vi "01TRM800.vi"() -> ()   [LabVIEW 2020]
uses:
  <vilib>/Instr/_visa.llb/VISA Configure Serial Port (Instr).vi
panel:
  out "error out":errorcluster
  out "String":string
  in  "stop":bool
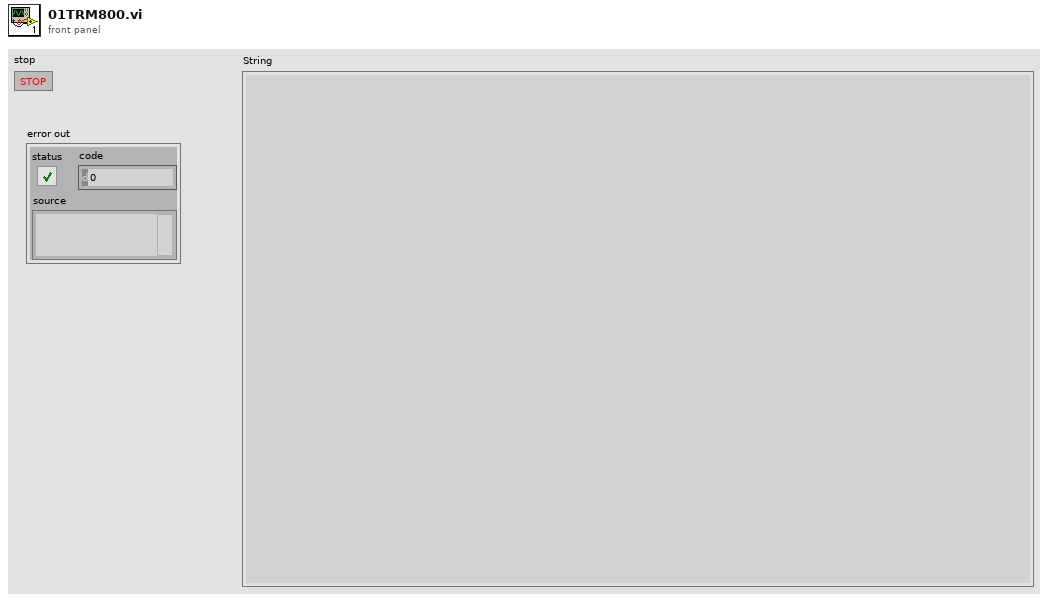
[diagram p1: front panel]
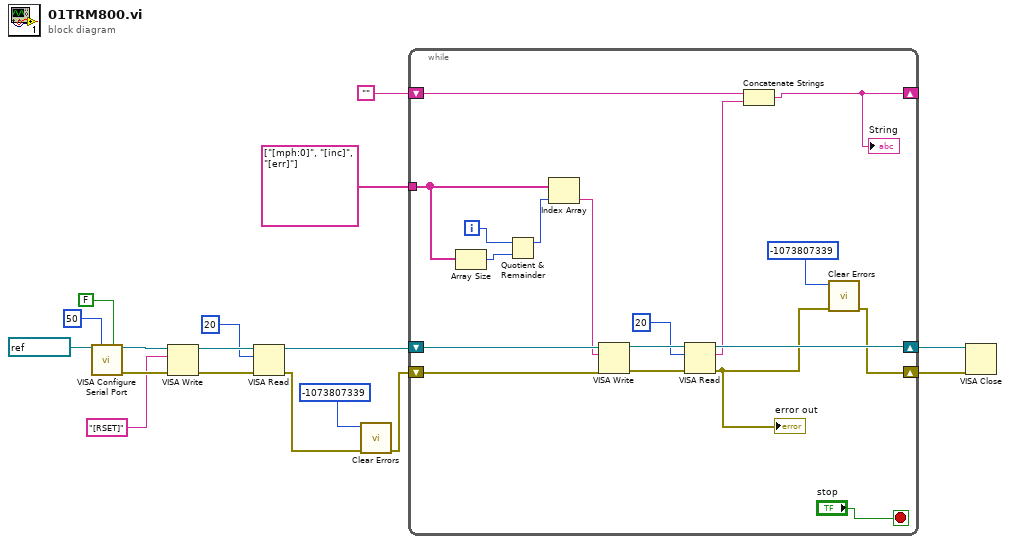
[diagram p0: block diagram]
diagram:
  n1 = call-poly "VISA Configure Serial Port"("VISA resource name"=refnum<visa-resource-name> "COM7", "timeout (10sec)"=u32 50, "Enable Termination\nChar (T)"=FALSE ("Enable Termination\nChar (T)")) -> ("VISA resource name out"=w7:refnum<visa-resource-name>, "error out"=w6:errorcluster)  [unwired: 11 in]
  n2 = VISA Write(VISA resource name=w7, write buffer="[RSET]", error in (no error)=w6) -> (VISA resource name out=w9:refnum<visa-resource-name>, error out=w10:errorcluster)  [unwired: 1 out]
  n3 = VISA Read(VISA resource name=w9, byte count=u32 20, error in (no error)=w10) -> (VISA resource name out=w5:refnum<visa-resource-name>, error out=w3:errorcluster)  [unwired: 2 out]
  n4 = call <vilib>:"Clear Errors.vi"("error in (no error)"=w3, "specific error code to clear (0: all)"=-1073807339) -> ("error out"=w2:errorcluster)  [unwired: 4 in, 1 out]
  n5 = while {
    shift-right: [w24] -> w13
    shift-left: w5 -> [w35]
    shift-right: [w22] -> w12
    shift-left: w2 -> [w30]
    tunnel: string[] ["[mph:0]", "[inc]", "[err]"] -> [w34]
    shift-right: [w18] -> _
    shift-left: "" -> [w20]
    i -> [w32]
    stop <- "stop" stop-if-true
    n6 = Array Size(array=w34) -> (size(s)=w33:i32)
    n7 = Quotient & Remainder(x=w32, y=w33) -> (x-y*floor(x/y)=w31:i32)  [unwired: 1 out]
    n8 = Index Array(array=w34, index=w31) -> (element=w29:string)
    n9 = VISA Write(VISA resource name=w35, write buffer=w29, error in (no error)=w30) -> (VISA resource name out=w26:refnum<visa-resource-name>, error out=w27:errorcluster)  [unwired: 1 out]
    n10 = VISA Read(VISA resource name=w26, byte count=u32 20, error in (no error)=w27) -> (VISA resource name out=w24:refnum<visa-resource-name>, read buffer=w19:string, error out=w23:errorcluster)  [unwired: 1 out]
    "error out" <- w23
    n11 = Concatenate Strings(w20, w19) -> (w18:string)
    "String" <- w18
    n12 = call <vilib>:"Clear Errors.vi"("error in (no error)"=w23, "specific error code to clear (0: all)"=-1073807339) -> ("error out"=w22:errorcluster)  [unwired: 4 in, 1 out]
  }
  n13 = VISA Close(VISA resource name=w13, error in (no error)=w12) -> ()  [unwired: 1 out]
